vi "TMCM351-getLimit.vi"(4 "错误输入":errorcluster caption="错误输入（无错误）", 6 "motor":u8(ring) items=["x", "y", "z"], 7 "com in":refnum<visa-resource-name>) -> (0 "错误输出":errorcluster, 1 "right limit":bool, 2 "left limit":bool, 3 "com out":refnum<visa-resource-name>)   [LabVIEW 2018]
uses:
  module_param.vi
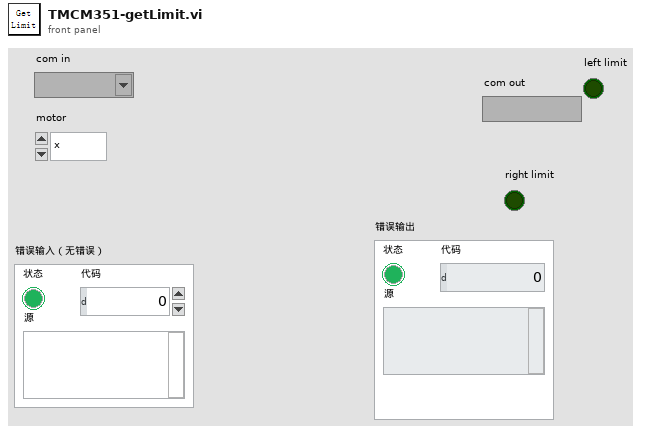
[diagram p1: front panel]
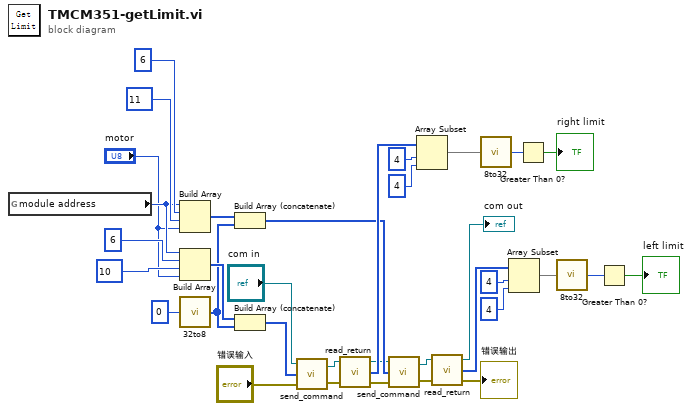
[diagram p0: block diagram]
diagram:
  n1 = global read "module_param.vi" "module address"() -> (w17:u8)
  n2 = Build Array(w17, u8 6, u8 11, "motor") -> (w15:u8[])
  n3 = Build Array(w17, u8 6, u8 10, "motor") -> (w32:u8[])
  n4 = call "32to8.vi"("32data_in"=0) -> ("8Array"=w14:u8[])
  n5 = Build Array (concatenate)(w15, w14) -> (w13:u8[])
  n6 = Build Array (concatenate)(w32, w14) -> (w31:u8[])
  n7 = call "send_command.vi"("错误输入"="错误输入", 3:w31, "com in"="com in") -> ("错误输出"=w28:errorcluster, "com out"=w29:refnum<visa-resource-name>)
  n8 = call "read_return.vi"("错误输入（无错误）"=w28, "com in"=w29) -> ("错误输出"=w11:errorcluster, "return out"=w26:u8[], "com out"=w12:refnum<visa-resource-name>)  [unwired: 1 in]
  n9 = call "send_command.vi"("错误输入"=w11, 3:w13, "com in"=w12) -> ("错误输出"=w9:errorcluster, "com out"=w10:refnum<visa-resource-name>)
  n10 = Array Subset(array=w26, index=4 ("索引"), length=4 ("长度")) -> (w23:u8[])
  n11 = call "read_return.vi"("错误输入（无错误）"=w9, "com in"=w10) -> ("错误输出"=→"错误输出":errorcluster, "return out"=w2:u8[], "com out"=→"com out":refnum<visa-resource-name>)  [unwired: 1 in]
  n12 = call "8to32.vi"("Arrayin"=w23) -> ("data32"=w22:i32)
  n13 = Array Subset(array=w2, index=4 ("索引"), length=4 ("长度")) -> (w4:u8[])
  n14 = Greater Than 0?(x=w22) -> (x > 0?=→"right limit":bool)
  n15 = call "8to32.vi"("Arrayin"=w4) -> ("data32"=w3:i32)
  n16 = Greater Than 0?(x=w3) -> (x > 0?=→"left limit":bool)
